vi "DIAdem Get Version.vi"(7 "error in (no error)":errorcluster, 10 "DIAdem Reference":T1) -> (0 "error out":errorcluster, 1 "Revision":i32, 2 "Version":i32, 3 "DIAdem Reference":T1)   [LabVIEW 2020]
doc: "This VI returns the version and revision of the DIAdem application. The version and revision are returned as integer values."
uses:
  <vilib>/ExportToExcel/DIAdem Reference.ctl
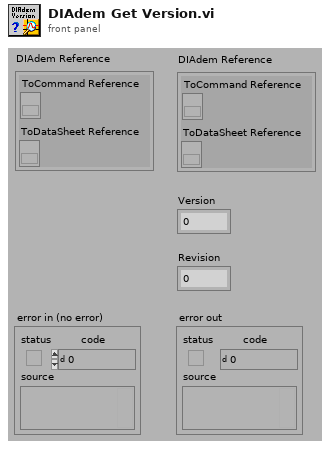
[diagram p1: front panel]
types:
  T1 = typedef "DIAdem Reference.ctl" = cluster{"ToCommand Reference":refnum<k7>, "ToDataSheet Reference":refnum<k7>}
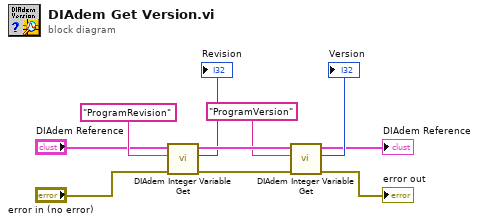
[diagram p0: block diagram]
diagram:
  n1 = call <vilib>:"DIAdem Integer Variable Get.vi"("error in (no error)"="error in (no error)", "Variable Name"="ProgramRevision", "DIAdem Reference"="DIAdem Reference") -> ("error out"=w7:errorcluster, "Value"=→"Revision":i32, "DIAdem Reference"=w6:T1)  [unwired: 6 in]
  n2 = call <vilib>:"DIAdem Integer Variable Get.vi"("error in (no error)"=w7, "Variable Name"="ProgramVersion", "DIAdem Reference"=w6) -> ("error out"=→"error out":errorcluster, "Value"=→"Version":i32, "DIAdem Reference"=→"DIAdem Reference":T1)  [unwired: 6 in]
